vi "WPI_DashboardProcessControlPacket.vi"(11 "data in":string) -> (3 "Control Info":T1)   [LabVIEW 2025]
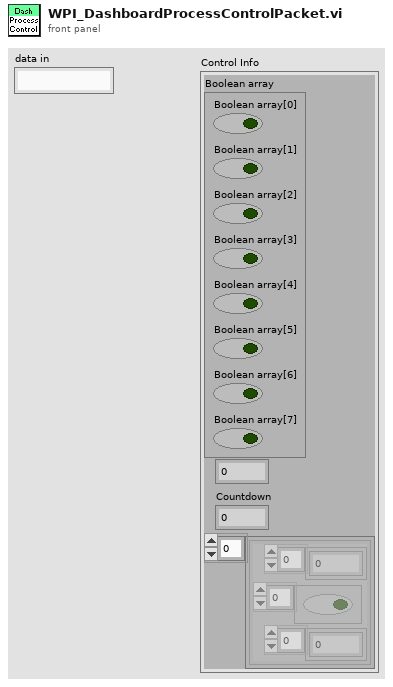
[diagram p1: front panel]
types:
  T1 = cluster{"Boolean array":cluster{"Boolean array[0]":bool, "Boolean array[1]":bool, "Boolean array[2]":bool, "Boolean array[3]":bool, "Boolean array[4]":bool, "Boolean array[5]":bool, "Boolean array[6]":bool, "Boolean array[7]":bool}, u8, "Countdown":sgl, cluster{dbl[], bool[], i16[]}[]}
  T2 = cluster{"packet # out":u16, "Version":u8, u8, u8, u8}
  T3 = cluster{"Boolean array[0]":bool, "Boolean array[1]":bool, "Boolean array[2]":bool, "Boolean array[3]":bool, "Boolean array[4]":bool, "Boolean array[5]":bool, "Boolean array[6]":bool, "Boolean array[7]":bool}
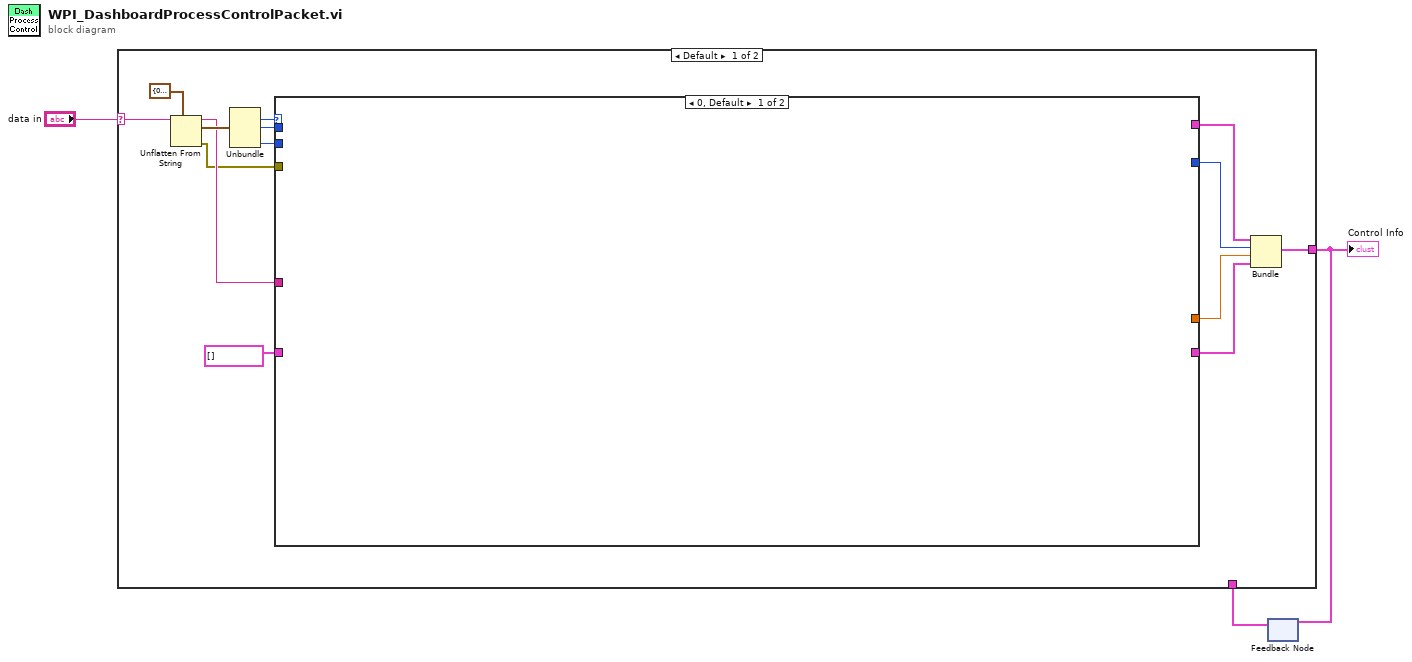
[diagram p0: block diagram]
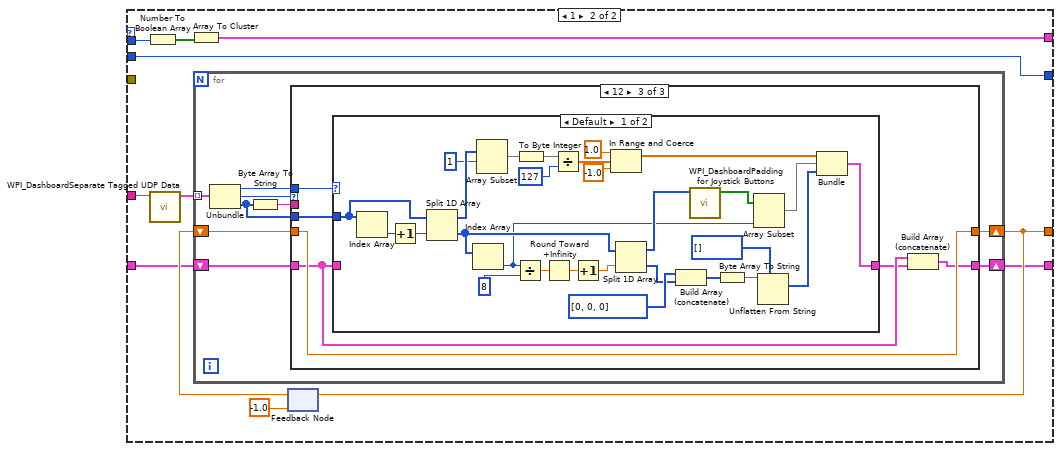
[diagram p2: hidden frame]
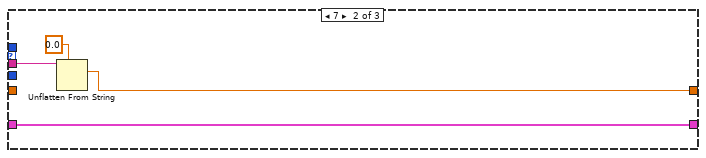
[diagram p4: hidden frame]
diagram:
  n1 = feedback #1() -> (w2:T1)  [unwired: 1 in]
  n2 = case shown="Default" "data in" {
    selector: "data in" -> [w4 _]
    tunnel: [w7 w78] -> w3
    tunnel: w2 -> [_ w78]
    frame Default {
      n3 = Unflatten From String(type=T2 {"packet # out"=0, "Version"=0, 0, 0, 0} ("output cluster"), binary string=w4) -> (rest of the binary string=w12:string, value=w16:T2, error out=w6:errorcluster)  [unwired: 1 in, 2 out]
      n4 = Unbundle(w16) -> ("Version"=w15:u8, w14:u8, w13:u8)  [unwired: 2 out]
      n5 = case shown="0, Default" w15 {
        tunnel: w14 -> [_ w28]
        tunnel: [_ w26] -> w11
        tunnel: [_ w25] -> w10
        tunnel: w13 -> [_ w25]
        tunnel: w12 -> [_ w24]
        tunnel: [_ w20] -> w9
        tunnel: [_ w19] -> w8
        tunnel: w6 -> [_ _]
        tunnel: cluster{dbl[], bool[], i16[]}[] [] -> [_ w18]
        frame 0, Default {
        }
        frame 1 {
          n6 = Number To Boolean Array(number=w28) -> (Boolean array=w27:bool[])
          n7 = call <vilib>:"WPI_DashboardSeparate Tagged UDP Data.vi"("String"=w24) -> ("Tagged Array"=w23:cluster{u8, u8, "unsigned byte array":u8[]}[])  [unwired: 10 in]
          n8 = Array To Cluster(array=w27) -> (cluster=w26:T3)
          n9 = feedback #2(sgl -1.0 ("Countdown")) -> (w21:sgl)
          n10 = for {
            tunnel: w23 -> [w37] mode=indexing
            shift-right: [w34] -> w20
            shift-left: w21 -> [w33]
            shift-right: [w30] -> w19
            shift-left: w18 -> [w29]
            n11 = Unbundle(w37) -> (w31:u8, w36:u8, "unsigned byte array"=w32:u8[])
            n12 = Byte Array To String(unsigned byte array=w32) -> (string=w35:string)
            n13 = case shown="12" w36 {
              tunnel: w35 -> [_ w43 _]
              tunnel: [w39 w41 w49] -> w34
              tunnel: w33 -> [w39 _ w49]
              tunnel: w32 -> [_ _ w47]
              tunnel: w31 -> [_ _ w48]
              tunnel: [w38 w40 w44] -> w30
              tunnel: w29 -> [w38 w40 w46]
              frame 0, Default {
              }
              frame 7 {
                n14 = Unflatten From String(type=sgl 0.0 ("Countdown"), binary string=w43) -> (value=w41:sgl)  [unwired: 3 in, 2 out]
              }
              frame 12 {
                n15 = case shown="Default" w48 {
                  tunnel: w47 -> [w76 _]
                  tunnel: [w50 _] -> w45
                  tunnel: w46 -> [_ _]
                  frame Default {
                    n16 = Index Array(array=w76) -> (element=w77:u8)  [unwired: 1 in]
                    n17 = Increment(x=w77) -> (x+1=w75:u8)
                    n18 = Split 1D Array(array=w76, index=w75) -> (first subarray=w73:u8[], second subarray=w74:u8[])
                    n19 = Index Array(array=w74) -> (element=w58:u8)  [unwired: 1 in]
                    n20 = Array Subset(array=w73, index=1) -> (w72:u8[])  [unwired: 1 in]
                    n21 = Divide(x=w58, y=8) -> (x/y=w62:dbl)
                    n22 = To Byte Integer(number=w72) -> (8bit integer=w66:i8[])
                    n23 = Round Toward +Infinity(x=w62) -> (ceil(x): smallest int >= x=w61:dbl)
                    n24 = Divide(x=w66, y=127) -> (x/y=w67:dbl[])
                    n25 = Increment(x=w61) -> (x+1=w60:dbl)
                    n26 = In Range and Coerce(upper limit=1.0, x=w67, lower limit=-1.0) -> (coerced(x)=w64:dbl[])  [unwired: 1 out]
                    n27 = Split 1D Array(array=w74, index=w60) -> (first subarray=w70:u8[], second subarray=w55:u8[])
                    n28 = Build Array (concatenate)(u8[] [0, 0, 0], w55) -> (w54:u8[])
                    n29 = call <vilib>:"WPI_DashboardPadding for Joystick Buttons.vi"("Array"=w70) -> ("Boolean array"=w59:bool[])  [unwired: 10 in]
                    n30 = Byte Array To String(unsigned byte array=w54) -> (string=w53:string)
                    n31 = Array Subset(array=w59, length=w58) -> (w57:bool[])  [unwired: 1 in]
                    n32 = Unflatten From String(type=i16[] [], binary string=w53) -> (value=w51:i16[])  [unwired: 3 in, 2 out]
                    n33 = Bundle(w64, w57, w51) -> (w50:cluster{dbl[], bool[], i16[]})  [unwired: 1 in]
                  }
                  frame 1 {
                  }
                }
                n34 = Build Array (concatenate)(w46, w45) -> (w44:cluster{dbl[], bool[], i16[]}[])
              }
            }
          }
          n35 = feedback-in #2(w20) -> ()
        }
      }
      n36 = Bundle("Boolean array"=w11, w10, "Countdown"=w9, w8) -> (w7:T1)  [unwired: 1 in]
    }
    frame "" {
    }
  }
  "Control Info" <- w3
  n37 = feedback-in #1(w3) -> ()
